vi "Get Last Log Info.vi"(8 "error in":errorcluster, 11 "CIF Message Type":T2) -> (0 "error out":errorcluster, 3 "Log Info":T1)   [LabVIEW 2021, in "CIFLogs.lvlib"]
uses:
  CIFLogs.lvlib
  Typedef/Message Type.ctl
  Typedef/Log Info.ctl
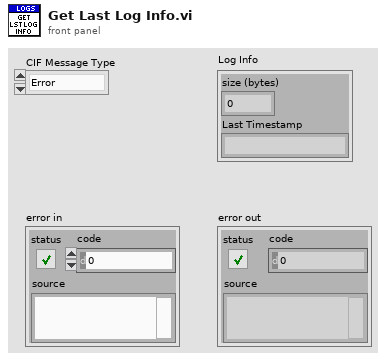
[diagram p1: front panel]
types:
  T1 = typedef "CIFLogs.lvlib/Log Info.ctl" = cluster{"size (bytes)":i64, "Last Timestamp":string}
  T2 = typedef "CIFLogs.lvlib/Message Type.ctl" = enum16{"Error", "Information", "Print Terminal", "Configuration"}
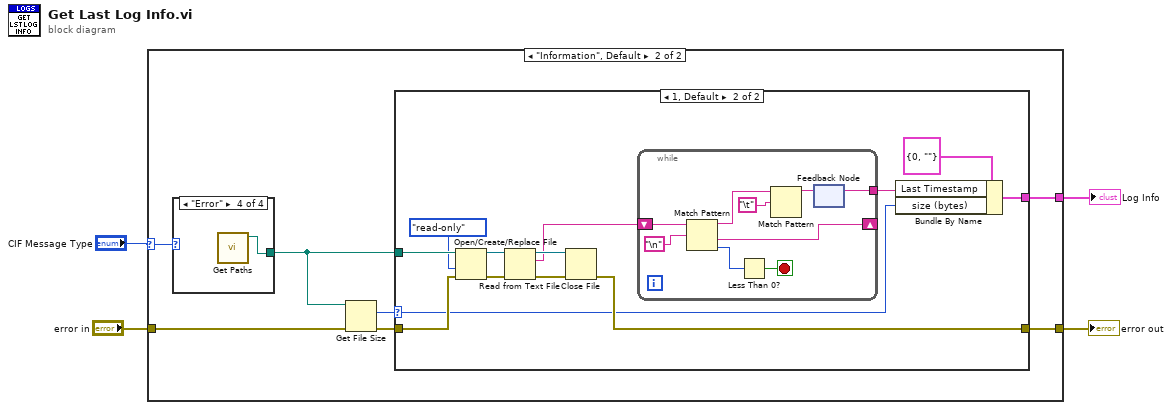
[diagram p0: block diagram]
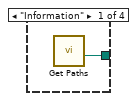
[diagram p4: hidden frame]
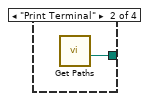
[diagram p5: hidden frame]
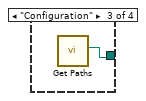
[diagram p6: hidden frame]
diagram:
  n1 = case shown="\"Information\", Default" "CIF Message Type" {
    selector: "CIF Message Type" -> [_ w11]
    tunnel: [_ w10] -> w3
    tunnel: "error in" -> [w5 w9]
    tunnel: [w5 w7] -> w1
    frame "Print Terminal" {
    }
    frame "Information", Default {
      n2 = case shown="\"Error\"" w11 {
        tunnel: [w36 w37 w38 w39] -> w12
        frame "Information" {
          n3 = call "Get Paths.vi"() -> ("Info Log"=w36:path)  [unwired: 9 in, 2 out]
        }
        frame "Print Terminal" {
          n4 = call "Get Paths.vi"() -> ("Info Log"=w37:path)  [unwired: 9 in, 2 out]
        }
        frame "Configuration" {
          n5 = call "Get Paths.vi"() -> ("Config Log"=w38:path)  [unwired: 9 in, 2 out]
        }
        frame "Error" {
          n6 = call "Get Paths.vi"() -> ("Error Log"=w39:path)  [unwired: 9 in, 2 out]
        }
      }
      n7 = Get File Size(file=w12, error in=w9) -> (size (in bytes)=w6:i64, 0:w8:errorcluster)  [unwired: 1 out]
      n8 = case shown="1, Default" w6 {
        selector: w6 -> [_ w15]
        tunnel: w12 -> [_ w21]
        tunnel: [_ w18] -> w10
        tunnel: w8 -> [w13 w17]
        tunnel: [w13 w16] -> w7
        frame 0 {
        }
        frame 1, Default {
          n9 = Open/Create/Replace File(file path (use dialog)=w21, error in=w17, access (0:read/write)=enum16{"read/write", "read-only", "write-only"}."read-only") -> (refnum out=w25:refnum<file>, error out=w24:errorcluster)  [unwired: 3 in, 1 out]
          n10 = Read from Text File(file (use dialog)=w25, error in=w24) -> (refnum out=w26:refnum<file>, text=w22:string, error out=w23:errorcluster)  [unwired: 2 in, 1 out]
          n11 = Close File(refnum=w26, error in=w23) -> (error out=w16:errorcluster)  [unwired: 1 out]
          n12 = while {
            shift-right: [w34] -> _
            shift-left: w22 -> [w35]
            tunnel: [w27] -> w19
            stop <- w32 stop-if-true
            n13 = Match Pattern(string=w35, regular expression="\n") -> (before substring=w31:string, after substring=w34:string, offset past match=w33:i32)  [unwired: 1 in, 1 out]
            n14 = Less Than 0?(x=w33) -> (x < 0?=w32:bool)
            n15 = Match Pattern(string=w31, regular expression="\t") -> (before substring=w28:string)  [unwired: 1 in, 3 out]
            n16 = feedback-in #1(w28) -> ()
            n17 = feedback #1() -> (w27:string)  [unwired: 1 in]
          }
          n18 = Bundle By Name(cluster=T1 {"size (bytes)"=0, "Last Timestamp"=""} ("Log Info 2"), "Last Timestamp"=w19, "size (bytes)"=w15) -> (w18:T1)
        }
      }
    }
  }
  "Log Info" <- w3
  "error out" <- w1
